vi "VI Tree.vi"   [LabVIEW 2015, in "Micron Optics sm130.lvlib"]
doc: "This is the instrument driver for the Micron Optics sm130. The VI Tree displays all the user-callable VIs of the instrument driver in an organized table."
uses:
  Micron Optics sm130.lvlib
panel:
  # "(c) 2009 - 2012 National Instruments.  ALL RIGHTS RESERVED."
  # "SEE DIAGRAM\nFOR VI TREE."
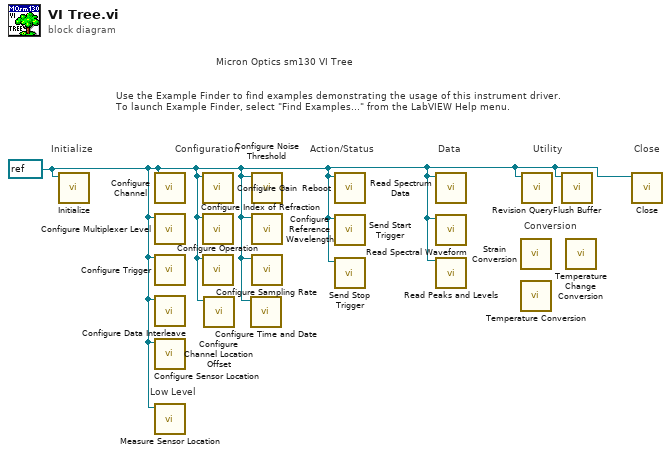
[diagram p0: block diagram]
diagram:
  w1 = refnum<visa-resource-name> refnum ("VISA resource name")
  # "Conversion"
  # "Micron Optics sm130 VI Tree"
  # "Low Level"
  # "Use the Example Finder to find examples demonstrating the usage of this instrument driver.\nTo launch Example Finder, select \"Find Examples...\" from the LabVIEW Help menu."
  # "Configuration"
  # "Utility"
  # "Data"
  # "Action/Status"
  # "Close"
  # "Initialize"
  n1 = call "Initialize.vi"("VISA resource name"=w1) -> ()  [unwired: 9 in, 2 out]
  n2 = call "Configure Channel.vi"("VISA resource name"=w1) -> ()  [unwired: 9 in, 2 out]
  n3 = call "Configure Multiplexer Level.vi"("VISA resource name"=w1) -> ()  [unwired: 9 in, 2 out]
  n4 = call "Configure Trigger.vi"("VISA resource name"=w1) -> ()  [unwired: 12 in, 3 out]
  n5 = call "Configure Data Interleave.vi"("VISA resource name"=w1) -> ()  [unwired: 9 in, 2 out]
  n6 = call "Configure Sensor Location.vi"("VISA resource name"=w1) -> ()  [unwired: 9 in, 2 out]
  n7 = call "Measure Sensor Location.vi"("VISA resource name"=w1) -> ()  [unwired: 9 in, 2 out]
  n8 = call "Configure Gain.vi"("VISA resource name"=w1) -> ()  [unwired: 9 in, 2 out]
  n9 = call "Configure Index of Refraction.vi"("VISA resource name"=w1) -> ()  [unwired: 9 in, 2 out]
  n10 = call "Configure Operation.vi"("VISA resource name"=w1) -> ()  [unwired: 9 in, 2 out]
  n11 = call "Configure Channel Location Offset.vi"("VISA resource name"=w1) -> ()  [unwired: 9 in, 2 out]
  n12 = call "Configure Time and Date.vi"("VISA resource name"=w1) -> ()  [unwired: 9 in, 2 out]
  n13 = call "Configure Noise Threshold.vi"("VISA resource name"=w1) -> ()  [unwired: 9 in, 2 out]
  n14 = call "Configure Reference Wavelength.vi"("VISA resource name"=w1) -> ()  [unwired: 9 in, 2 out]
  n15 = call "Configure Sampling Rate.vi"("VISA resource name"=w1) -> ()  [unwired: 9 in, 2 out]
  n16 = call "Reboot.vi"("VISA resource name"=w1) -> ()  [unwired: 9 in, 2 out]
  n17 = call "Send Start Trigger.vi"("VISA resource name"=w1) -> ()  [unwired: 9 in, 2 out]
  n18 = call "Send Stop Trigger.vi"("VISA resource name"=w1) -> ()  [unwired: 9 in, 2 out]
  n19 = call "Read Spectrum Data.vi"("VISA resource name"=w1) -> ()  [unwired: 6 in, 5 out]
  n20 = call "Read Spectral Waveform.vi"("VISA resource name"=w1) -> ()  [unwired: 8 in, 3 out]
  n21 = call "Read Peaks and Levels.vi"("VISA resource name"=w1) -> ()  [unwired: 6 in, 9 out]
  n22 = call "Strain Conversion.vi"() -> ()  [unwired: 15 in, 1 out]
  n23 = call "Temperature Conversion.vi"() -> ()  [unwired: 11 in, 1 out]
  n24 = call "Revision Query.vi"("VISA resource name"=w1) -> ()  [unwired: 7 in, 4 out]
  n25 = call "Flush Buffer.vi"("VISA resource name"=w1) -> ()  [unwired: 9 in, 2 out]
  n26 = call "Temperature Change Conversion.vi"() -> ()  [unwired: 11 in, 1 out]
  n27 = call "Close.vi"("VISA resource name"=w1) -> ()  [unwired: 10 in, 1 out]
